vi "initIP.vi"(3 "error in":errorcluster, 4 "IP Address":string="010000000000", 5 "reference in":refnum<visa-resource-name>) -> (0 "error out":errorcluster, 1 "初始化状态":bool, 2 "reference out":refnum<visa-resource-name>)   [LabVIEW 2010]
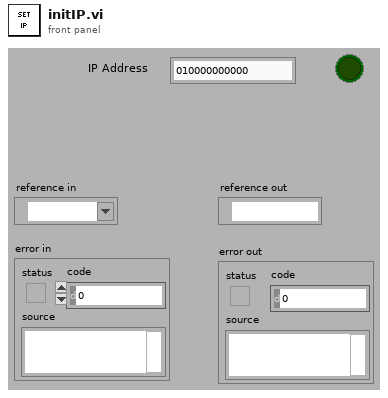
[diagram p1: front panel]
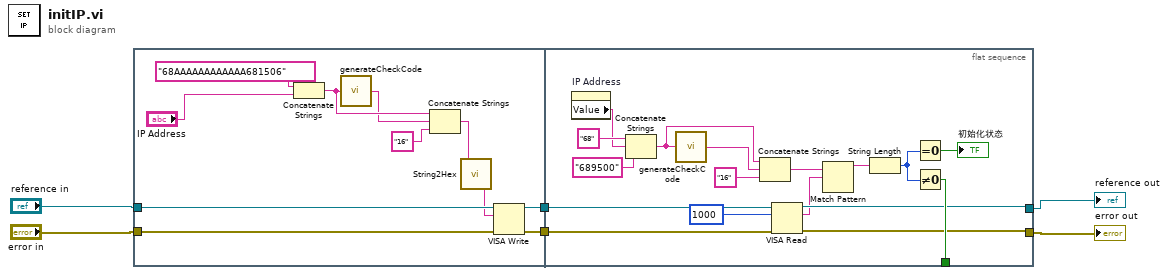
[diagram p0: block diagram]
diagram:
  n1 = flat-sequence {
    tunnel: "reference in" -> [w14]
    tunnel: "error in" -> [w13]
    tunnel: [w11] -> w6
    tunnel: [w10] -> w5
    tunnel: w6 -> [w23]
    tunnel: w5 -> [w21]
    tunnel: [w25] -> _
    tunnel: [w19] -> w2
    tunnel: [w20] -> w1
    frame #0 {
      n2 = Concatenate Strings("68AAAAAAAAAAAA681506", "IP Address") -> (w17:string)
      n3 = call "generateCheckCode.vi"("Data"=w17) -> ("CheckCode"=w15:string)
      n4 = Concatenate Strings(w17, w15, "16" ("字符串")) -> (w12:string)
      n5 = call "String2Hex.vi"("value"=w12) -> ("String"=w7:string)
      n6 = VISA Write(VISA resource name=w14, write buffer=w7, error in (no error)=w13) -> (VISA resource name out=w11:refnum<visa-resource-name>, error out=w10:errorcluster)  [unwired: 1 out]
    }
    frame #1 {
      n7 = property on="IP Address" class="Str"() -> ("Value"=w26:string)  [unwired: 2 in, 2 out]
      n8 = Concatenate Strings("68" ("字符串"), w26, "689500" ("字符串")) -> (w27:string)
      n9 = call "generateCheckCode.vi"("Data"=w27) -> ("CheckCode"=w32:string)
      n10 = Concatenate Strings(w27, w32, "16" ("字符串")) -> (w34:string)
      n11 = VISA Read(VISA resource name=w23, byte count=u32 1000 ("字节总数"), error in (no error)=w21) -> (VISA resource name out=w19:refnum<visa-resource-name>, read buffer=w18:string, error out=w20:errorcluster)  [unwired: 1 out]
      n12 = Match Pattern(string=w34, regular expression=w18) -> (before substring=w29:string)  [unwired: 1 in, 3 out]
      n13 = String Length(string=w29) -> (length=w30:i32)
      n14 = Equal To 0?(x=w30) -> (x = 0?=→"初始化状态":bool)
      n15 = Not Equal To 0?(x=w30) -> (x != 0?=w25:bool)
    }
  }
  "error out" <- w1
  "reference out" <- w2
